vi "Test Configure.vi"(0 "Template Tx Test in":refnum<class "niDTS Calibration Cal Execute RF Test.lvclass">, 11 "error in (no error)":errorcluster) -> (4 "Template Tx Test out":refnum<class "niDTS Calibration Cal Execute RF Test.lvclass">, 15 "error out":errorcluster)   [LabVIEW 2015, in "niDTS Utilities.lvlib" / "niDTS Calibration Cal Execute RF Test.lvclass"]
uses:
  niDTS Calibration Cal Execute RF Test.lvclass
  RiviInstDriver/InstDriver/Objects/InstDriver.lvclass/InstDriver.ctl
  niDTS Calibration Cal Execute RF Test.lvclass/niDTS Calibration Cal Execute RF Test.ctl
  RiviInstDriver/InstDriver/Objects/Read VISA resource.vi
  Properties/Calibration Cal Execute Set InstDriver Handle in.vi
  Properties/Calibration Cal Execute RF Test Set Ports.vi
  TestStand/Station/Objects/SystemTechnologyCatalog/niDTS SystemTechnologyCatalog.lvclass
  TestStand/Station/Objects/SystemDut/niDTS SystemDut.lvclass
  TestStand/niDTS TestStand.lvlib
  RiviInstDriver/niRfGeneralSettings/Objects/niRfGeneralSettings.lvclass
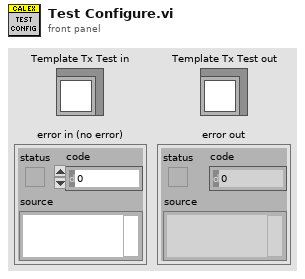
[diagram p1: front panel]
types:
  T1 = typedef "InstDriver.lvclass/niInstDriver INC Handle.ctl" = refnum<data-value>
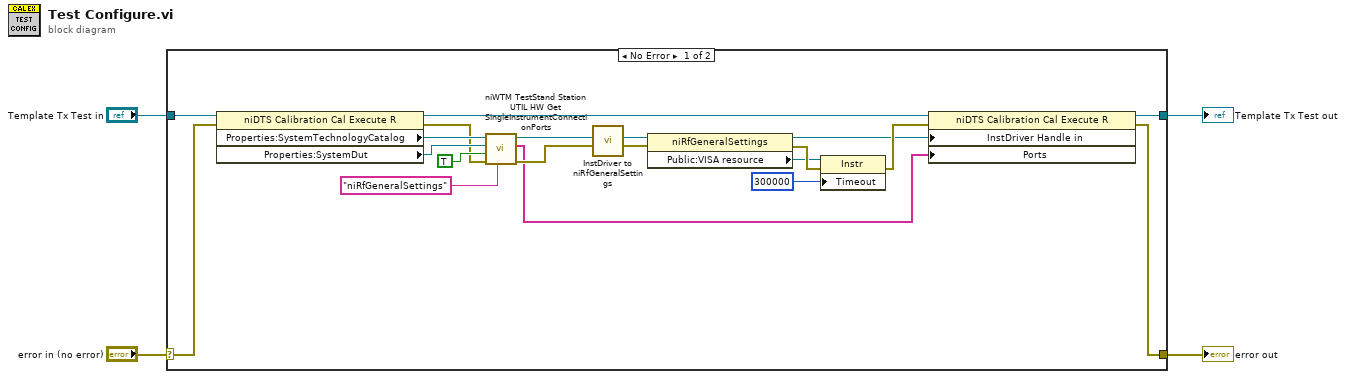
[diagram p0: block diagram]
diagram:
  n1 = case shown="No Error" "error in (no error)" {
    selector: "error in (no error)" -> [w20 w26]
    tunnel: [w19 w26] -> w3
    tunnel: "Template Tx Test in" -> [w18 w25]
    tunnel: [w17 w25] -> w1
    frame No Error {
      n2 = property class="niDTS Calibration Cal Execute R"(reference=w18, error in=w20) -> (reference out=w13:refnum<class "niDTS Calibration Cal Execute RF Test.lvclass">, error out=w21:errorcluster, "Properties:SystemTechnologyCatalog"=w24:refnum<class "niDTS SystemTechnologyCatalog.lvclass">, "Properties:SystemDut"=w23:refnum<class "niDTS SystemDut.lvclass">)
      n3 = call "niWTM TestStand Station UTIL HW Get SingleInstrumentConnectionPorts.vi"("InstDriver Name"="niRfGeneralSettings", "error in (no error)"=w21, "TX Instrument"=TRUE, "SystemDut"=w23, "SystemTechnologyCatalog"=w24) -> ("error out"=w14:errorcluster, "Ports"=w6:string[], "InstDriver Handle"=w15:T1)  [unwired: 4 in]
      n4 = call "InstDriver to niRfGeneralSettings.vi"("error in (no error)"=w14, "InstDriver Handle in"=w15) -> ("error out"=w11:errorcluster, "InstDriver Handle out"=w12:refnum<data-value>)  [unwired: 8 in]
      n5 = property class="niRfGeneralSettings"(reference=w12, error in=w11) -> (reference out=w5:refnum<data-value>, error out=w10:errorcluster, "Public:VISA resource"=w9:refnum<visa-resource-name>)
      n6 = property class="Instr"(reference=w9, error in=w10, "Timeout"=u32 300000 ("General Settings:Timeout Value")) -> (error out=w7:errorcluster)  [unwired: 1 out]
      n7 = property class="niDTS Calibration Cal Execute R"(reference=w13, error in=w7, "InstDriver Handle in"=w5, "Ports"=w6) -> (reference out=w17:refnum<class "niDTS Calibration Cal Execute RF Test.lvclass">, error out=w19:errorcluster)
    }
    frame Error {
    }
  }
  "error out" <- w3
  "Template Tx Test out" <- w1
